vi "move2.vi"(1 "CAM_Control":T1, 2 "dist(mm)":dbl) -> (0 "MoveString":string)   [LabVIEW 2019]
panel:
  out "number":i32
  out "array":bool[](array[boolean])
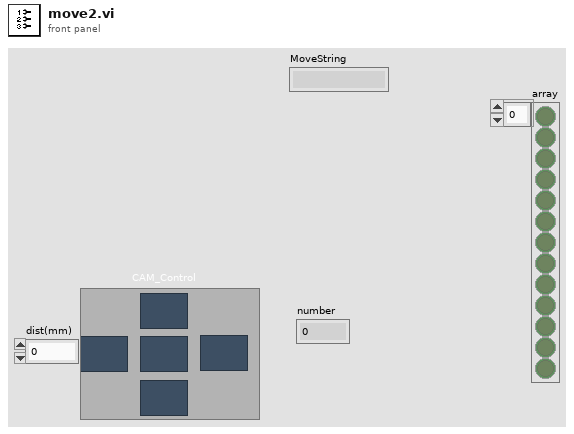
[diagram p1: front panel]
types:
  T1 = cluster{"Back Button":bool, "Forward Button":bool, "Up Button":bool, "Down Button":bool, "Reset Button":bool}
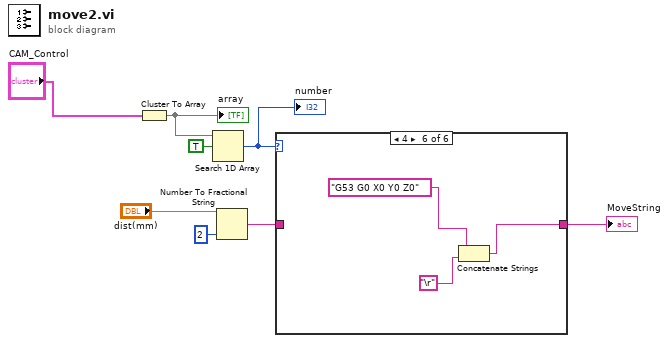
[diagram p0: block diagram]
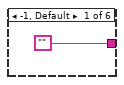
[diagram p2: hidden frame]
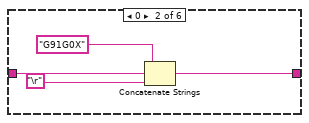
[diagram p3: hidden frame]
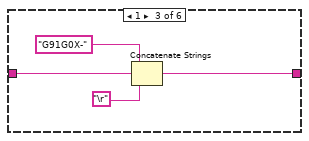
[diagram p4: hidden frame]
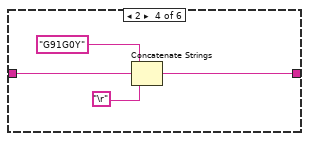
[diagram p5: hidden frame]
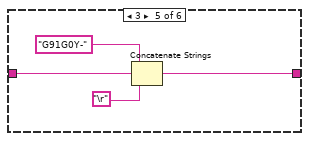
[diagram p6: hidden frame]
diagram:
  n1 = Cluster To Array(cluster="CAM_Control") -> (array=w8:bool[])
  "array" <- w8
  n2 = Search 1D Array(1D array=w8, element=TRUE) -> (index of element=w6:i32)  [unwired: 1 in]
  "number" <- w6
  n3 = Number To Fractional String(number="dist(mm)", precision (6)=i16 2) -> (F-format string=w3:string)  [unwired: 2 in]
  n4 = case shown="4" w6 {
    tunnel: w3 -> [_ w11 w16 w20 w24 _]
    tunnel: ["" w12 w14 w18 w22 w26] -> w2
    frame -1, Default {
    }
    frame 0 {
      n5 = Concatenate Strings("G91G0X", w11, "\r") -> (w12:string)
    }
    frame 1 {
      n6 = Concatenate Strings("G91G0X-", w16, "\r") -> (w14:string)
    }
    frame 2 {
      n7 = Concatenate Strings("G91G0Y", w20, "\r") -> (w18:string)
    }
    frame 3 {
      n8 = Concatenate Strings("G91G0Y-", w24, "\r") -> (w22:string)
    }
    frame 4 {
      n9 = Concatenate Strings("G53 G0 X0 Y0 Z0" ("Command 2"), "\r") -> (w26:string)
    }
  }
  "MoveString" <- w2
